vi "CreateClassHeirachy.vi"(8 "error in (no error)":errorcluster, 11 "Application in":refnum<class "Application.lvclass">) -> (0 "error out":errorcluster, 3 "Application out":refnum<class "Application.lvclass">)   [LabVIEW 2020, in "Mermaid.lvlib" / "Application.lvclass"]
uses:
  Application.lvclass
  _Interface/Interface.lvclass
  _Class/Class.lvclass
  Application.lvclass/Application.ctl
panel:
  out "Int":string
  out "Parent":string
  out "Child":string
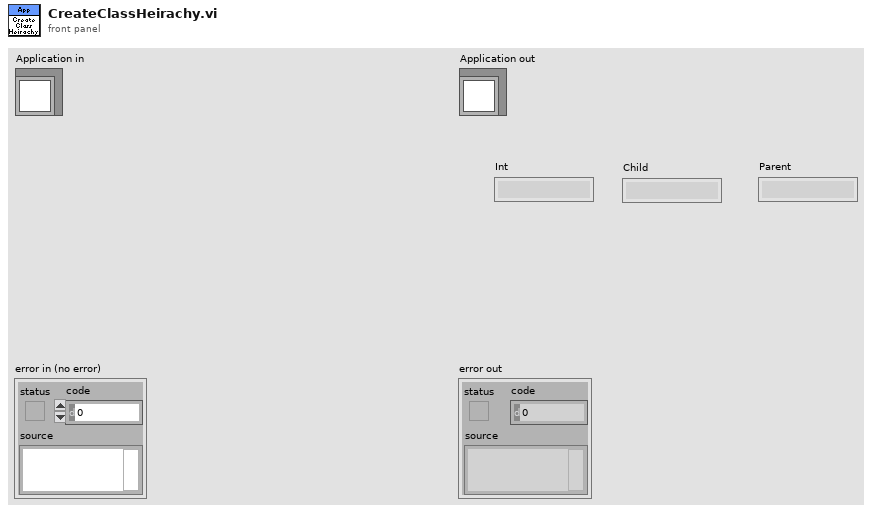
[diagram p1: front panel]
types:
  T1 = typedef "Mermaid.lvlib/ParseMermaid.lvclass/ClassData.ctl" = cluster{"Name":string, "ClassType":T2, "PublicMethods":string[], "PrivateMethods":string[], "FinalPublicAttributes":T3, "FinalPrivateAttributes":T3, "Parent":string}
  T2 = typedef "Mermaid.lvlib/ParseMermaid.lvclass/ClassType.ctl" = enum16{"Interface", "Class"}
  T3 = typedef "Mermaid.lvlib/ParseMermaid.lvclass/Attributes.ctl" = cluster{"Name":string, "Type":i32}[]
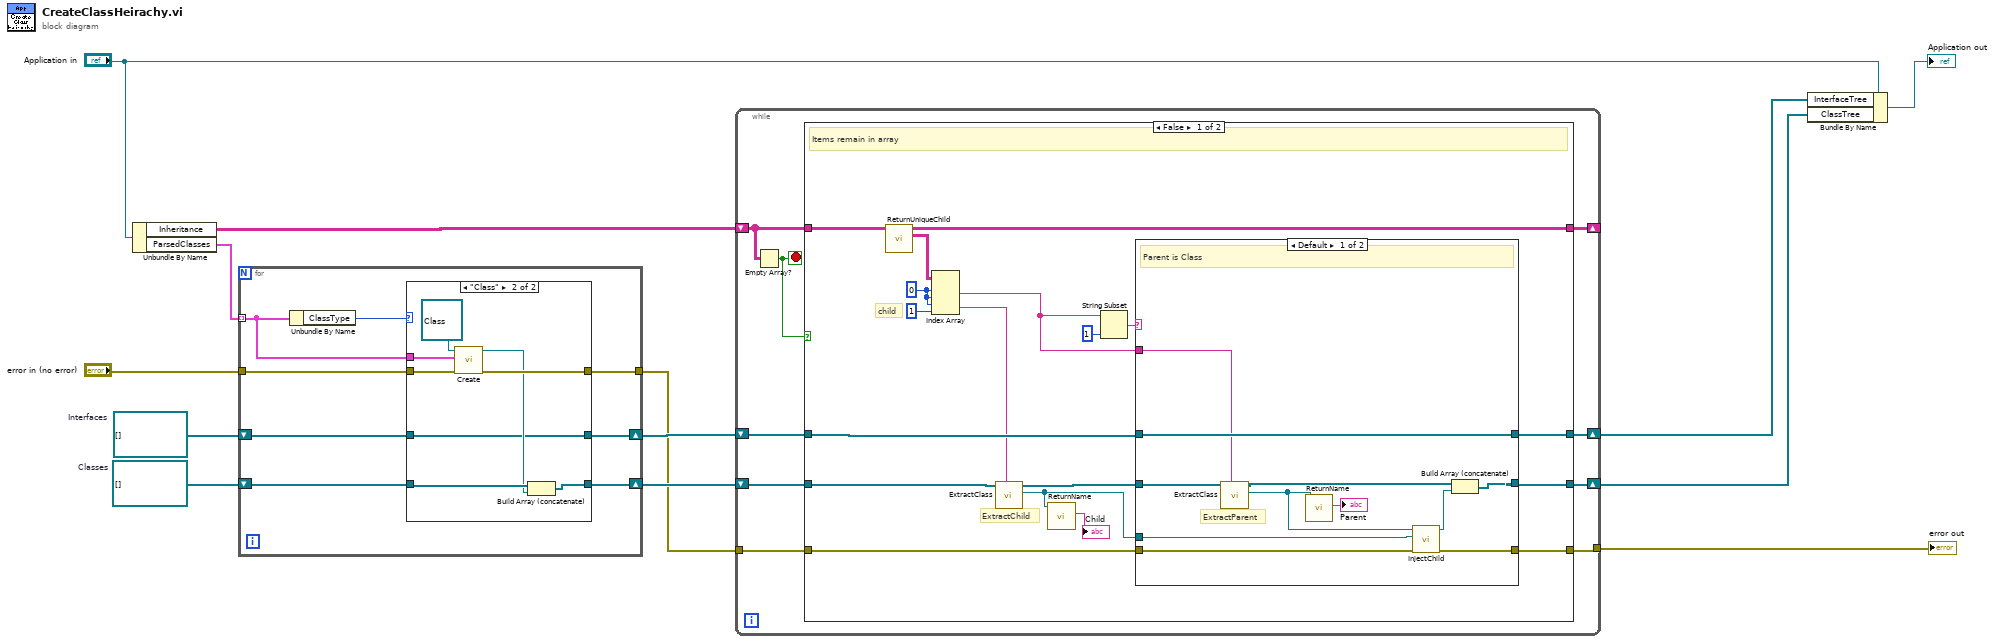
[diagram p0: block diagram]
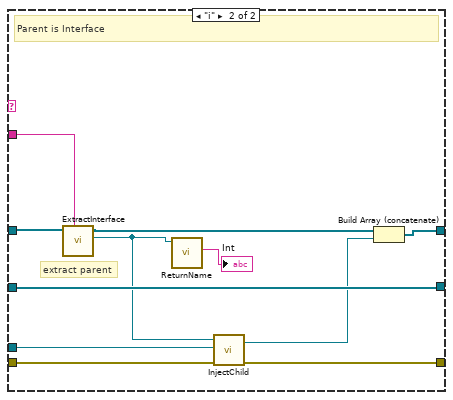
[diagram p2: hidden frame]
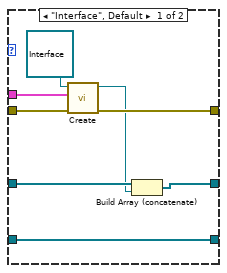
[diagram p4: hidden frame]
diagram:
  w10 = refnum<class "Class.lvclass">[] []  # Classes
  w11 = refnum<class "Interface.lvclass">[] []  # Interfaces
  n1 = Unbundle By Name("Application in") -> ("Inheritance"=w7:string[][], "ParsedClasses"=w13:T1[])
  n2 = for {
    tunnel: w13 -> [w20] mode=indexing
    tunnel: "error in (no error)" -> [w19]
    tunnel: [w18] -> w4
    shift-right: [w14] -> w6
    shift-left: w11 -> [w15]
    shift-right: [w16] -> w5
    shift-left: w10 -> [w17]
    n3 = Unbundle By Name(w20) -> ("ClassType"=w21:T2)
    n4 = case shown="\"Class\"" w21 {
      tunnel: w20 -> [w27 w36]
      tunnel: w19 -> [w29 w37]
      tunnel: [w28 w34] -> w18
      tunnel: w17 -> [w25 w33]
      tunnel: [w25 w31] -> w16
      tunnel: w15 -> [w24 w30]
      tunnel: [w22 w30] -> w14
      frame "Interface", Default {
        n5 = call-dynamic "Create.vi"("error in (no error)"=w29, "Class"=w27, "Interface In"=refnum<class "Interface.lvclass"> refnum) -> ("error out"=w28:errorcluster, "Interface out"=w23:refnum<class "Interface.lvclass">)  [unwired: 7 in]
        n6 = Build Array (concatenate)(w24, w23) -> (w22:refnum<class "Interface.lvclass">[])
      }
      frame "Class" {
        n7 = call-dynamic "Create.vi"("error in (no error)"=w37, "Class"=w36, "Class In"=refnum<class "Class.lvclass"> refnum) -> ("error out"=w34:errorcluster, "Class out"=w32:refnum<class "Class.lvclass">)  [unwired: 7 in]
        n8 = Build Array (concatenate)(w33, w32) -> (w31:refnum<class "Class.lvclass">[])
      }
    }
  }
  n9 = while {
    shift-right: [w46] -> _
    shift-left: w7 -> [w45]
    shift-right: [w40] -> w3
    shift-left: w6 -> [w41]
    shift-right: [w42] -> w2
    shift-left: w5 -> [w43]
    tunnel: w4 -> [w39]
    tunnel: [w38] -> w1
    stop <- w44 stop-if-true
    n10 = Empty Array?(array=w45) -> (empty?=w44:bool)
    n11 = case shown="False" w44 {
      tunnel: w45 -> [w58 w90]
      tunnel: [w48 w90] -> w46
      tunnel: w43 -> [w64 w89]
      tunnel: [w63 w89] -> w42
      tunnel: w41 -> [w62 w88]
      tunnel: [w61 w88] -> w40
      tunnel: w39 -> [w60 w87]
      tunnel: [w59 w87] -> w38
      frame False {
        w52 = 0 ("index (row)")
        # "child"
        # "ExtractChild"
        # "Items remain in array"
        n12 = call "ReturnUniqueChild.vi"("Array In"=w58) -> ("Unique Child"=w47:string[][], "Array Out"=w48:string[][])  [unwired: 9 in]
        n13 = Index Array(array=w47, index (row) #1=w52, index (col) #1=w52, index (row) #2=w52, index (col) #2=1 ("disabled index (col)")) -> (element #1=w49:string, element #2=w50:string)
        n14 = call "ExtractClass.vi"("String"=w50, "Array in"=w64) -> ("ClassOut"=w54:refnum<class "Class.lvclass">, "ArrayOut"=w55:refnum<class "Class.lvclass">[])  [unwired: 8 in]
        n15 = call-dynamic "ReturnName.vi"("Class in"=w54) -> ("Name"=→"Child":string)  [unwired: 8 in, 2 out]
        n16 = String Subset(string=w49, length (rest)=1 ("length (rest)")) -> (substring=w56:string)  [unwired: 1 in]
        n17 = case shown="Default" w56 {
          tunnel: w55 -> [w71 w86]
          tunnel: w49 -> [w65 w76]
          tunnel: w54 -> [w75 w79]
          tunnel: [w74 w86] -> w63
          tunnel: w62 -> [w73 w83]
          tunnel: [w73 w85] -> w61
          tunnel: w60 -> [w70 w81]
          tunnel: [w72 w84] -> w59
          frame Default {
            # "ExtractParent"
            # "Parent is Class"
            n18 = call "ExtractClass.vi"("String"=w65, "Array in"=w71) -> ("ClassOut"=w67:refnum<class "Class.lvclass">, "ArrayOut"=w69:refnum<class "Class.lvclass">[])  [unwired: 8 in]
            n19 = call-dynamic "ReturnName.vi"("Class in"=w67) -> ("Name"=→"Parent":string)  [unwired: 8 in, 2 out]
            n20 = call-dynamic "InjectChild.vi"("error in (no error)"=w70, "Child"=w75, "Class in"=w67) -> ("error out"=w72:errorcluster, "Class out"=w68:refnum<class "Class.lvclass">)  [unwired: 7 in]
            n21 = Build Array (concatenate)(w69, w68) -> (w74:refnum<class "Class.lvclass">[])
          }
          frame "i" {
            # "extract parent"
            # "Parent is Interface"
            n22 = call "ExtractInterface.vi"("String"=w76, "Array in"=w83) -> ("InterfaceOut"=w78:refnum<class "Interface.lvclass">, "ArrayOut"=w82:refnum<class "Interface.lvclass">[])  [unwired: 8 in]
            n23 = call-dynamic "ReturnName.vi"("Interface in"=w78) -> ("Name"=→"Int":string)  [unwired: 8 in, 2 out]
            n24 = call-dynamic "InjectChild.vi"("error in (no error)"=w81, "Child"=w79, "Interface in"=w78) -> ("error out"=w84:errorcluster, "Interface out"=w80:refnum<class "Interface.lvclass">)  [unwired: 7 in]
            n25 = Build Array (concatenate)(w82, w80) -> (w85:refnum<class "Interface.lvclass">[])
          }
        }
      }
      frame True {
        # "Empty Array"
      }
    }
  }
  "error out" <- w1
  n26 = Bundle By Name(cluster="Application in", "InterfaceTree"=w3, "ClassTree"=w2) -> (→"Application out":refnum<class "Application.lvclass">)
